vi "GetPolarAndR.vi"(10 "all rows 3":dbl[][](array[numeric])) -> (2 "Array 2":dbl[](array[numeric]), 3 "Array":dbl[](array[numeric]))   [LabVIEW 2018]
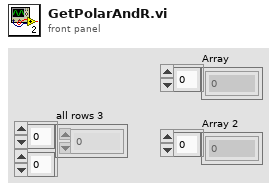
[diagram p1: front panel]
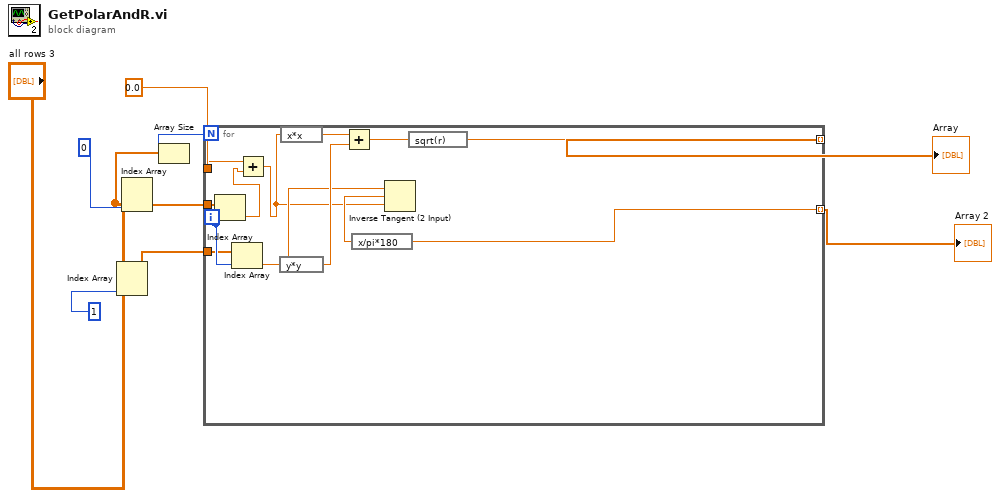
[diagram p0: block diagram]
diagram:
  n1 = Index Array(array="all rows 3", index (col)=1 ("disabled index (col)")) -> (element=w6:dbl[])  [unwired: 1 in]
  n2 = Index Array(array="all rows 3", index (col)=0 ("disabled index (col)")) -> (element=w5:dbl[])  [unwired: 1 in]
  n3 = Array Size(array=w5) -> (size(s)=w3:i32)
  n4 = for {
    N: w3 -> [_]
    tunnel: w5 -> [w22]
    tunnel: w6 -> [w18]
    tunnel: [w14] -> w7 mode=indexing
    tunnel: [w13] -> w8 mode=indexing
    tunnel: 0.0 ("x") -> [w10]
    i -> [w19]
    n5 = Index Array(array=w22, index=w19) -> (element=w12:dbl)
    n6 = Index Array(array=w18, index=w19) -> (element=w15:dbl)
    n7 = Add(x=w10, y=w12) -> (x+y=w11:dbl)
    n8 = expression code="y*y"(w15) -> (w17:dbl)
    n9 = expression code="x*x"(w11) -> (w20:dbl)
    n10 = Add(x=w20, y=w17) -> (x+y=w21:dbl)
    n11 = Inverse Tangent (2 Input)(1:w11, 2:w15) -> (0:w16:dbl)
    n12 = expression code="x/pi*180"(w16) -> (w14:dbl)
    n13 = expression code="sqrt(r)"(w21) -> (w13:dbl)
  }
  "Array 2" <- w7
  "Array" <- w8
